vi "get_node_ids.vi"(11 "edge":refnum<class "Edge.lvclass">) -> (1 "sink-id":refnum<class "ID.lvclass">, 2 "source-id":refnum<class "ID.lvclass">)   [LabVIEW 2020, in "graph.lvlib" / "Edge.lvclass"]
uses:
  Edge.lvclass
  ID/ID.lvclass
  Edge.lvclass/Edge.ctl
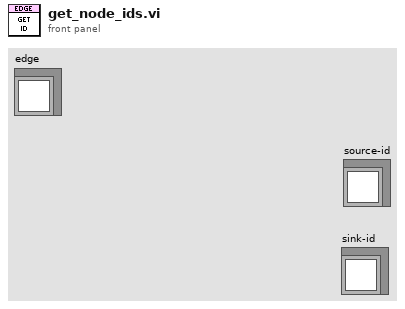
[diagram p1: front panel]
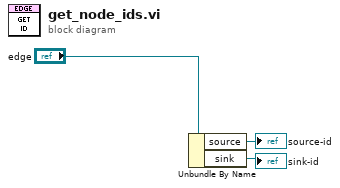
[diagram p0: block diagram]
diagram:
  n1 = Unbundle By Name("edge") -> ("source"=→"source-id":refnum<class "ID.lvclass">, "sink"=→"sink-id":refnum<class "ID.lvclass">)
